vi "CRYGoto Cursor.vi"(7 "sOption":string, 8 "Active Cursor":u32, 10 "Graph Ref":refnum<vi>, 11 "Graph Type":string) -> ()   [LabVIEW 2013]
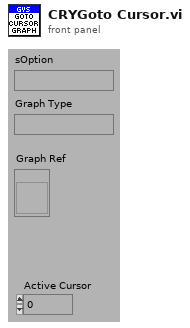
[diagram p1: front panel]
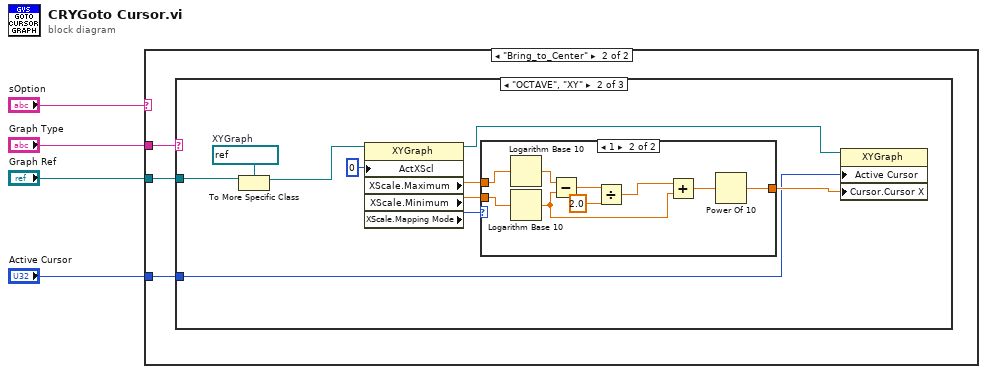
[diagram p0: block diagram]
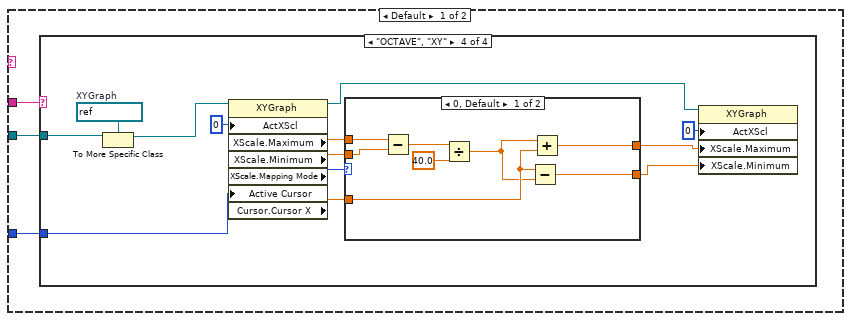
[diagram p2: hidden frame]
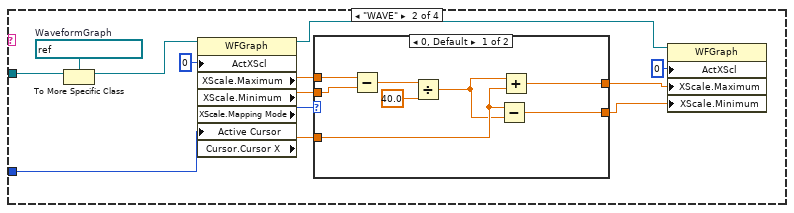
[diagram p4: hidden frame]
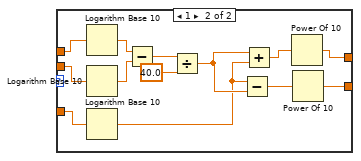
[diagram p5: hidden frame]
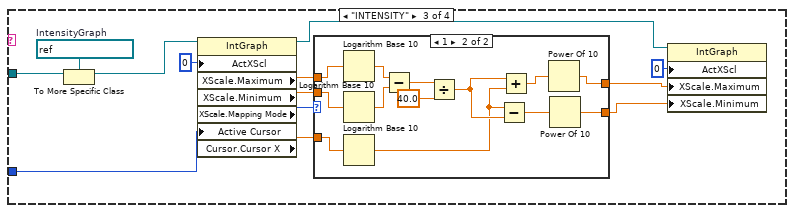
[diagram p6: hidden frame]
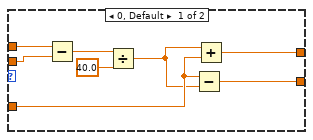
[diagram p7: hidden frame]
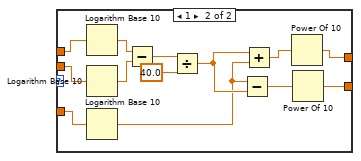
[diagram p8: hidden frame]
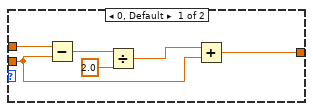
[diagram p10: hidden frame]
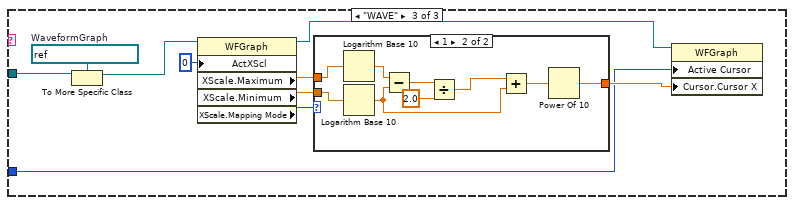
[diagram p11: hidden frame]
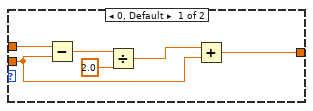
[diagram p12: hidden frame]
diagram:
  n1 = case shown="\"Bring_to_Center\"" "sOption" {
    tunnel: "Graph Type" -> [w7 w112]
    tunnel: "Active Cursor" -> [w6 w111]
    tunnel: "Graph Ref" -> [w5 w110]
    frame Default {
      n2 = case shown="\"OCTAVE\", \"XY\"" w7 {
        tunnel: w6 -> [_ w16 w50 w84]
        tunnel: w5 -> [_ w10 w44 w77]
        frame Default {
        }
        frame "WAVE" {
          w9 = refnum<vi> refnum  # WaveformGraph
          n3 = To More Specific Class(target class=w9, reference=w10) -> (specific class reference=w8:refnum<vi>)  [unwired: 1 in, 1 out]
          n4 = property on="Property Node" class="WFGraph"(reference=w8, "ActXScl"=0 ("Active X Scale"), "Active Cursor"=w16) -> (reference out=w14:refnum<vi>, "XScale.Maximum"=w20:dbl, "XScale.Minimum"=w19:dbl, "XScale.Mapping Mode"=w17:u8, "Cursor.Cursor X"=w15:dbl)  [unwired: 1 in, 1 out]
          n5 = case shown="0, Default" w17 {
            tunnel: w20 -> [w25 w37]
            tunnel: w19 -> [w28 w38]
            tunnel: [w21 w31] -> w12
            tunnel: [w24 w29] -> w11
            tunnel: w15 -> [w23 w34]
            frame 0, Default {
              n6 = Subtract(x=w25, y=w28) -> (x-y=w27:dbl)
              n7 = Divide(x=w27, y=40.0) -> (x/y=w22:dbl)
              n8 = Subtract(x=w23, y=w22) -> (x-y=w24:dbl)
              n9 = Add(x=w22, y=w23) -> (x+y=w21:dbl)
            }
            frame 1 {
              n10 = Logarithm Base 10(1:w37) -> (0:w36:dbl)
              n11 = Logarithm Base 10(1:w38) -> (0:w35:dbl)
              n12 = Logarithm Base 10(1:w34) -> (0:w33:dbl)
              n13 = Subtract(x=w36, y=w35) -> (x-y=w41:dbl)
              n14 = Divide(x=w41, y=40.0) -> (x/y=w39:dbl)
              n15 = Subtract(x=w33, y=w39) -> (x-y=w30:dbl)
              n16 = Add(x=w39, y=w33) -> (x+y=w32:dbl)
              n17 = Power Of 10(x=w32) -> (10^x=w31:dbl)
              n18 = Power Of 10(x=w30) -> (10^x=w29:dbl)
            }
          }
          n19 = property on="Property Node" class="WFGraph"(reference=w14, "ActXScl"=0 ("Active X Scale"), "XScale.Maximum"=w12, "XScale.Minimum"=w11) -> ()  [unwired: 1 in, 2 out]
        }
        frame "INTENSITY" {
          w43 = refnum<vi> refnum  # IntensityGraph
          n20 = To More Specific Class(target class=w43, reference=w44) -> (specific class reference=w42:refnum<vi>)  [unwired: 1 in, 1 out]
          n21 = property on="Property Node" class="IntGraph"(reference=w42, "ActXScl"=0 ("Active X Scale"), "Active Cursor"=w50) -> (reference out=w48:refnum<vi>, "XScale.Maximum"=w54:dbl, "XScale.Minimum"=w53:dbl, "XScale.Mapping Mode"=w51:u8, "Cursor.Cursor X"=w49:dbl)  [unwired: 1 in, 1 out]
          n22 = case shown="1" w51 {
            tunnel: w54 -> [w59 w71]
            tunnel: w53 -> [w62 w72]
            tunnel: [w55 w65] -> w46
            tunnel: [w58 w63] -> w45
            tunnel: w49 -> [w57 w68]
            frame 0, Default {
              n23 = Subtract(x=w59, y=w62) -> (x-y=w61:dbl)
              n24 = Divide(x=w61, y=40.0) -> (x/y=w56:dbl)
              n25 = Subtract(x=w57, y=w56) -> (x-y=w58:dbl)
              n26 = Add(x=w56, y=w57) -> (x+y=w55:dbl)
            }
            frame 1 {
              n27 = Logarithm Base 10(1:w71) -> (0:w70:dbl)
              n28 = Logarithm Base 10(1:w72) -> (0:w69:dbl)
              n29 = Logarithm Base 10(1:w68) -> (0:w67:dbl)
              n30 = Subtract(x=w70, y=w69) -> (x-y=w75:dbl)
              n31 = Divide(x=w75, y=40.0) -> (x/y=w73:dbl)
              n32 = Subtract(x=w67, y=w73) -> (x-y=w64:dbl)
              n33 = Add(x=w73, y=w67) -> (x+y=w66:dbl)
              n34 = Power Of 10(x=w66) -> (10^x=w65:dbl)
              n35 = Power Of 10(x=w64) -> (10^x=w63:dbl)
            }
          }
          n36 = property on="Property Node" class="IntGraph"(reference=w48, "ActXScl"=0 ("Active X Scale"), "XScale.Maximum"=w46, "XScale.Minimum"=w45) -> ()  [unwired: 1 in, 2 out]
        }
        frame "OCTAVE", "XY" {
          w78 = refnum<vi> refnum  # XYGraph
          n37 = To More Specific Class(target class=w78, reference=w77) -> (specific class reference=w76:refnum<vi>)  [unwired: 1 in, 1 out]
          n38 = property on="Property Node" class="XYGraph"(reference=w76, "ActXScl"=0 ("Active X Scale"), "Active Cursor"=w84) -> (reference out=w82:refnum<vi>, "XScale.Maximum"=w88:dbl, "XScale.Minimum"=w87:dbl, "XScale.Mapping Mode"=w85:u8, "Cursor.Cursor X"=w83:dbl)  [unwired: 1 in, 1 out]
          n39 = case shown="0, Default" w85 {
            tunnel: w88 -> [w93 w105]
            tunnel: w87 -> [w96 w106]
            tunnel: [w89 w99] -> w80
            tunnel: [w92 w97] -> w79
            tunnel: w83 -> [w91 w102]
            frame 0, Default {
              n40 = Subtract(x=w93, y=w96) -> (x-y=w95:dbl)
              n41 = Divide(x=w95, y=40.0) -> (x/y=w90:dbl)
              n42 = Subtract(x=w91, y=w90) -> (x-y=w92:dbl)
              n43 = Add(x=w90, y=w91) -> (x+y=w89:dbl)
            }
            frame 1 {
              n44 = Logarithm Base 10(1:w105) -> (0:w104:dbl)
              n45 = Logarithm Base 10(1:w106) -> (0:w103:dbl)
              n46 = Logarithm Base 10(1:w102) -> (0:w101:dbl)
              n47 = Subtract(x=w104, y=w103) -> (x-y=w109:dbl)
              n48 = Divide(x=w109, y=40.0) -> (x/y=w107:dbl)
              n49 = Subtract(x=w101, y=w107) -> (x-y=w98:dbl)
              n50 = Add(x=w107, y=w101) -> (x+y=w100:dbl)
              n51 = Power Of 10(x=w100) -> (10^x=w99:dbl)
              n52 = Power Of 10(x=w98) -> (10^x=w97:dbl)
            }
          }
          n53 = property on="Property Node" class="XYGraph"(reference=w82, "ActXScl"=0 ("Active X Scale"), "XScale.Maximum"=w80, "XScale.Minimum"=w79) -> ()  [unwired: 1 in, 2 out]
        }
      }
    }
    frame "Bring_to_Center" {
      n54 = case shown="\"OCTAVE\", \"XY\"" w112 {
        tunnel: w111 -> [_ w113 w139]
        tunnel: w110 -> [_ w115 w141]
        frame Default {
        }
        frame "OCTAVE", "XY" {
          w116 = refnum<vi> refnum  # XYGraph
          n55 = To More Specific Class(target class=w116, reference=w115) -> (specific class reference=w114:refnum<vi>)  [unwired: 1 in, 1 out]
          n56 = property on="Property Node" class="XYGraph"(reference=w114, "ActXScl"=0 ("Active X Scale")) -> (reference out=w118:refnum<vi>, "XScale.Maximum"=w122:dbl, "XScale.Minimum"=w121:dbl, "XScale.Mapping Mode"=w119:u8)  [unwired: 1 in, 1 out]
          n57 = case shown="1" w119 {
            tunnel: w122 -> [w126 w134]
            tunnel: w121 -> [w123 w130]
            tunnel: [w124 w131] -> w117
            frame 0, Default {
              n58 = Subtract(x=w126, y=w123) -> (x-y=w128:dbl)
              n59 = Divide(x=w128, y=2.0) -> (x/y=w125:dbl)
              n60 = Add(x=w125, y=w123) -> (x+y=w124:dbl)
            }
            frame 1 {
              n61 = Logarithm Base 10(1:w134) -> (0:w133:dbl)
              n62 = Logarithm Base 10(1:w130) -> (0:w129:dbl)
              n63 = Subtract(x=w133, y=w129) -> (x-y=w137:dbl)
              n64 = Divide(x=w137, y=2.0) -> (x/y=w135:dbl)
              n65 = Add(x=w135, y=w129) -> (x+y=w132:dbl)
              n66 = Power Of 10(x=w132) -> (10^x=w131:dbl)
            }
          }
          n67 = property on="Property Node" class="XYGraph"(reference=w118, "Active Cursor"=w113, "Cursor.Cursor X"=w117) -> ()  [unwired: 1 in, 2 out]
        }
        frame "WAVE" {
          w138 = refnum<vi> refnum  # WaveformGraph
          n68 = To More Specific Class(target class=w138, reference=w141) -> (specific class reference=w140:refnum<vi>)  [unwired: 1 in, 1 out]
          n69 = property on="Property Node" class="WFGraph"(reference=w140, "ActXScl"=0 ("Active X Scale")) -> (reference out=w143:refnum<vi>, "XScale.Maximum"=w147:dbl, "XScale.Minimum"=w146:dbl, "XScale.Mapping Mode"=w144:u8)  [unwired: 1 in, 1 out]
          n70 = case shown="1" w144 {
            tunnel: w147 -> [w151 w159]
            tunnel: w146 -> [w148 w155]
            tunnel: [w149 w156] -> w142
            frame 0, Default {
              n71 = Subtract(x=w151, y=w148) -> (x-y=w153:dbl)
              n72 = Divide(x=w153, y=2.0) -> (x/y=w150:dbl)
              n73 = Add(x=w150, y=w148) -> (x+y=w149:dbl)
            }
            frame 1 {
              n74 = Logarithm Base 10(1:w159) -> (0:w158:dbl)
              n75 = Logarithm Base 10(1:w155) -> (0:w154:dbl)
              n76 = Subtract(x=w158, y=w154) -> (x-y=w162:dbl)
              n77 = Divide(x=w162, y=2.0) -> (x/y=w160:dbl)
              n78 = Add(x=w160, y=w154) -> (x+y=w157:dbl)
              n79 = Power Of 10(x=w157) -> (10^x=w156:dbl)
            }
          }
          n80 = property on="Property Node" class="WFGraph"(reference=w143, "Active Cursor"=w139, "Cursor.Cursor X"=w142) -> ()  [unwired: 1 in, 2 out]
        }
      }
    }
  }
